vi "MetaPushScript.vi"(11 "MetaScript":string) -> ()   [LabVIEW 2019]
panel:
  out "error out":errorcluster
  in  "error in (no error)":errorcluster
  in  "stop":bool
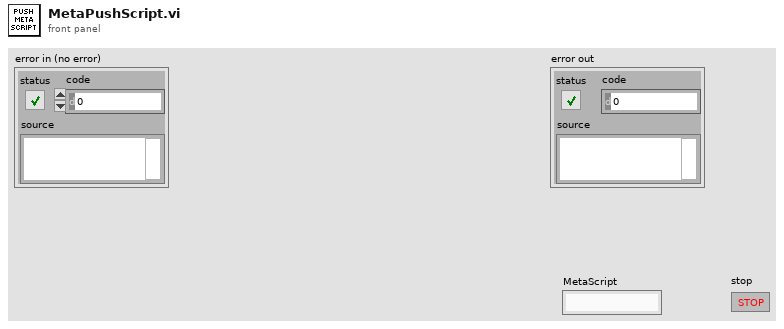
[diagram p1: front panel]
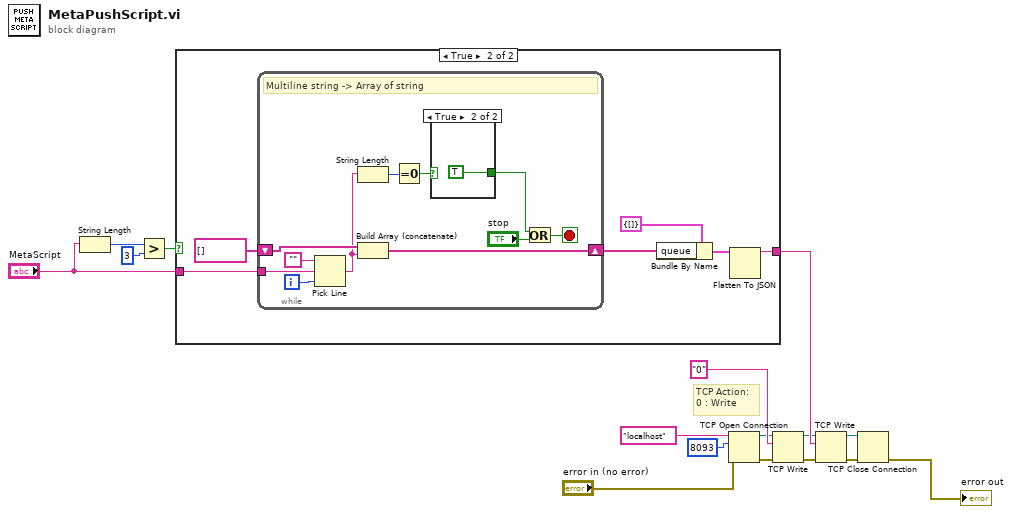
[diagram p0: block diagram]
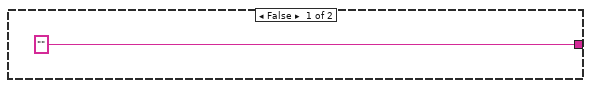
[diagram p2: hidden frame]
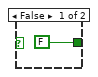
[diagram p3: hidden frame]
diagram:
  # "TCP Action:\n0 : Write"
  n1 = String Length(string="MetaScript") -> (length=w5:i32)
  n2 = Greater?(x=w5, y=3) -> (0:w4:bool)
  n3 = case shown="True" w4 {
    tunnel: "MetaScript" -> [_ w23]
    tunnel: ["" ("JSON string") w18] -> w16
    frame False {
    }
    frame True {
      n4 = while {
        shift-right: [w32] -> w21
        shift-left: string[] [] -> [w33]
        tunnel: w23 -> [w24]
        i -> [w34]
        stop <- w25 stop-if-true
        # "Multiline string -> Array of string"
        n5 = Pick Line(string ("")="", multi-line string=w24, line index=w34) -> (output string=w30:string)
        n6 = String Length(string=w30) -> (length=w29:i32)
        n7 = Build Array (concatenate)(w33, w30) -> (w32:string[])
        n8 = Equal To 0?(x=w29) -> (x = 0?=w28:bool)
        n9 = case shown="True" w28 {
          tunnel: [FALSE TRUE] -> w27
          frame False {
          }
          frame True {
          }
        }
        n10 = Or(x=w27, y="stop") -> (x .or. y?=w25:bool)
      }
      n11 = Bundle By Name(cluster=cluster{"queue":string[]} {"queue"=[]}, "queue"=w21) -> (w19:cluster{"queue":string[]})
      n12 = Flatten To JSON(anything=w19) -> (JSON string=w18:string)  [unwired: 2 in, 1 out]
    }
  }
  n13 = TCP Open Connection(address="localhost", remote port or service name=u16 8093, error in (no error)="error in (no error)") -> (connection ID=w9:refnum<k5>, error out=w8:errorcluster)  [unwired: 2 in]
  n14 = TCP Write(connection ID=w9, data in="0", error in (no error)=w8) -> (connection ID out=w12:refnum<k5>, error out=w7:errorcluster)  [unwired: 1 in, 1 out]
  n15 = TCP Write(connection ID=w12, data in=w16, error in (no error)=w7) -> (connection ID out=w11:refnum<k5>, error out=w10:errorcluster)  [unwired: 1 in, 1 out]
  n16 = TCP Close Connection(connection ID=w11, error in (no error)=w10) -> (error out=→"error out":errorcluster)  [unwired: 1 in, 1 out]
